vi "Find All Zeroes Inner Part (VI).vi"(6 "data":variant, 7 "f(x)":T1, 8 "error in":i32, 9 "accuracy":dbl=1e-08 format="%.2e", 10 "algorithm":u16, 11 "X and Y values":cluster{"X Values":dbl[], "Y Values":dbl[]} {"Y Values" format="%.2f"; "X Values" format="%.2f"}) -> (0 "error out":i32, 2 "f(Zeroes)":dbl[](array[numeric]) format="%.2f", 3 "Zeroes":dbl[](array[numeric]) format="%.2f")   [LabVIEW 2017, in "NI_Gmath.lvlib"]
uses:
  <vilib>/gmath/NI_Gmath.lvlib
  <vilib>/gmath/_ref_NR.llb/functionRefnum.ctl
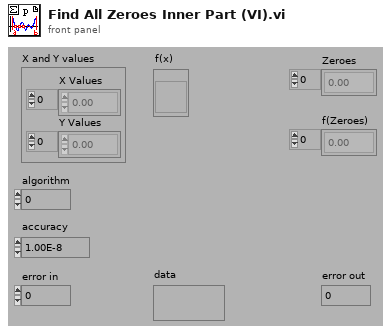
[diagram p1: front panel]
types:
  T1 = typedef "NI_Gmath.lvlib/functionRefnum.ctl" = refnum<vi>
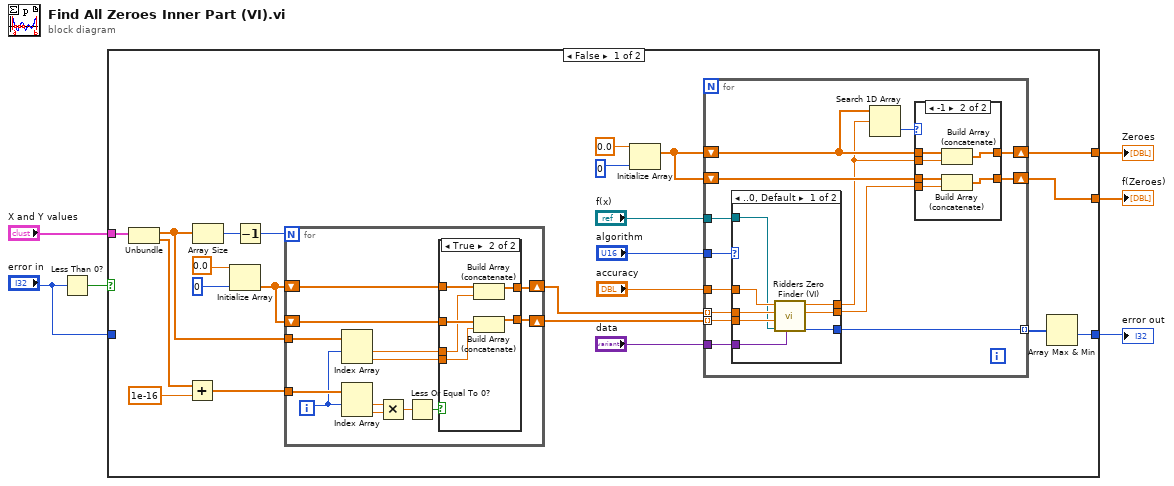
[diagram p0: block diagram]
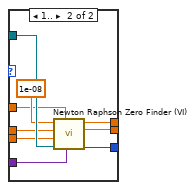
[diagram p3: hidden frame]
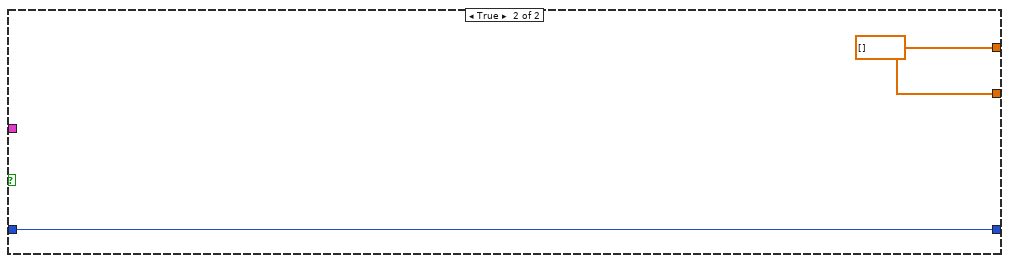
[diagram p5: hidden frame]
diagram:
  n1 = Less Than 0?(x="error in") -> (x < 0?=w2:bool)
  n2 = case shown="False" w2 {
    tunnel: "X and Y values" -> [w20 _]
    tunnel: [w11 w90] -> w5
    tunnel: [w10 w90] -> w4
    tunnel: [w9 w91] -> w3
    tunnel: "error in" -> [_ w91]
    frame False {
      n3 = Unbundle(w20) -> ("X Values"=w29:dbl[], "Y Values"=w23:dbl[])
      n4 = Add(x=w23, y=1e-16) -> (x+y=w25:dbl[])
      n5 = Array Size(array=w29) -> (size(s)=w21:i32)
      n6 = Initialize Array(0.0, 0) -> (w28:dbl[])
      n7 = Decrement(x=w21) -> (x-1=w22:i32)
      n8 = for {
        N: w22 -> [_]
        tunnel: w25 -> [w72]
        shift-right: [w78] -> w15
        shift-left: w28 -> [w79]
        shift-right: [w76] -> w14
        shift-left: w28 -> [w77]
        tunnel: w29 -> [w75]
        i -> [w69]
        n9 = Index Array(array=w75, index #1=w69) -> (element #1=w74:dbl, element #2=w73:dbl)  [unwired: 1 in]
        n10 = Index Array(array=w72, index #1=w69) -> (element #1=w71:dbl, element #2=w70:dbl)  [unwired: 1 in]
        n11 = Multiply(x=w71, y=w70) -> (x*y=w81:dbl)
        n12 = Less Or Equal To 0?(x=w81) -> (x <= 0?=w80:bool)
        n13 = case shown="True" w80 {
          tunnel: w79 -> [w83 w89]
          tunnel: [w83 w88] -> w78
          tunnel: w77 -> [w82 w87]
          tunnel: [w82 w86] -> w76
          tunnel: w74 -> [_ w85]
          tunnel: w73 -> [_ w84]
          frame False {
          }
          frame True {
            n14 = Build Array (concatenate)(w89, w85) -> (w88:dbl[])
            n15 = Build Array (concatenate)(w87, w84) -> (w86:dbl[])
          }
        }
      }
      n16 = Initialize Array(0.0, 0) -> (w18:dbl[])
      n17 = for {
        tunnel: w15 -> [w39] mode=indexing
        tunnel: w14 -> [w38] mode=indexing
        tunnel: "accuracy" -> [w37]
        shift-right: [w41] -> w11
        shift-left: w18 -> [w31]
        shift-right: [w42] -> w10
        shift-left: w18 -> [w43]
        tunnel: "algorithm" -> [w36]
        tunnel: [w35] -> w19 mode=indexing
        tunnel: "f(x)" -> [w34]
        tunnel: "data" -> [w33]
        n18 = case shown="..0, Default" w36 {
          tunnel: w37 -> [w59 w62]
          tunnel: w38 -> [w57 w60]
          tunnel: w39 -> [w58 w61]
          tunnel: [w54 w66] -> w40
          tunnel: [w55 w67] -> w30
          tunnel: [w56 w65] -> w35
          tunnel: w34 -> [w52 w64]
          tunnel: w33 -> [w53 w68]
          frame ..0, Default {
            n19 = call <vilib>:"Ridders Zero Finder (VI).vi"("data"=w53, "f(x)"=w52, "end"=w57, "start"=w58, "accuracy"=w59) -> ("error"=w56:i32, "f(zero)"=w54:dbl, "zero"=w55:dbl)  [unwired: 1 in, 3 out]
          }
          frame 1.. {
            n20 = call <vilib>:"Newton Raphson Zero Finder (VI).vi"("data"=w68, "accuracy"=w62, "f(x)"=w64, "end"=w60, "start"=w61, "h"=1e-08) -> ("error"=w65:i32, "f(zero)"=w66:dbl, "zero"=w67:dbl)  [unwired: 3 out]
          }
        }
        n21 = Search 1D Array(1D array=w31, element=w30) -> (index of element=w32:i32)  [unwired: 1 in]
        n22 = case shown="-1" w32 {
          tunnel: w31 -> [w45 w51]
          tunnel: w43 -> [w44 w50]
          tunnel: [w44 w49] -> w42
          tunnel: [w45 w48] -> w41
          tunnel: w30 -> [_ w47]
          tunnel: w40 -> [_ w46]
          frame 0, Default {
          }
          frame -1 {
            n23 = Build Array (concatenate)(w51, w47) -> (w48:dbl[])
            n24 = Build Array (concatenate)(w50, w46) -> (w49:dbl[])
          }
        }
      }
      n25 = Array Max & Min(array=w19) -> (min value=w9:i32)  [unwired: 3 out]
    }
    frame True {
      w90 = dbl[] []
    }
  }
  "error out" <- w3
  "f(Zeroes)" <- w4
  "Zeroes" <- w5
